vi "cached_threshold.vi"(1 "index":u8, 2 "cur_index":u8, 3 "new_val":fxp<+/-,32,16>) -> (0 "$_val":fxp<+/-,32,16>)   [LabVIEW 2018]
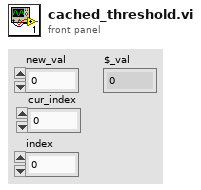
[diagram p1: front panel]
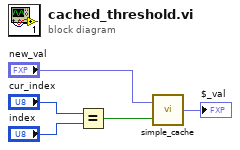
[diagram p0: block diagram]
diagram:
  n1 = Equal?(x="cur_index", y="index") -> (x = y?=w5:bool)
  n2 = call "simple_cache.vi"("refresh"=w5, "new_val"="new_val") -> ("$_val"=→"$_val":fxp<+/-,32,16>)
